vi "get_control_data.vi"(1 "DS Occurrence":refnum<k4>) -> ()   [LabVIEW 2011]
uses:
  <vilib>/Rock Robotics/WPI/Joystick/WPI_JoystickButtonState.ctl
  robot_control.ctl
  match_data.ctl
  <vilib>/Rock Robotics/WPI/DriverStation/WPI_DriverStationMatch Info.ctl
  <vilib>/Rock Robotics/WPI/DriverStation/WPI_DriverStationDerivedRobotMode.ctl
  <vilib>/Rock Robotics/WPI/DriverStation/WPI_DriverStationRobotMode.ctl
  Robot Global Data.vi
panel:
  in  "reinitialize":bool
  out "i per ms":dbl
  out "iterations":i32
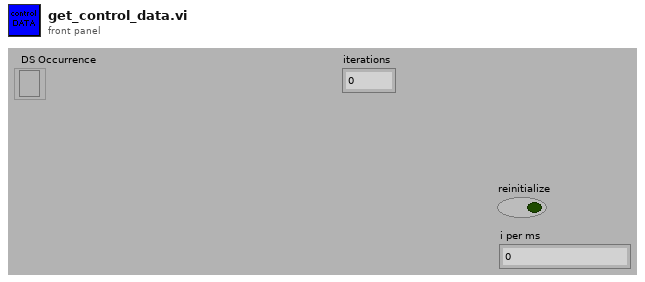
[diagram p1: front panel]
types:
  T1 = cluster{"Driver Station Digital Input (1-8)[0]":bool, "Driver Station Digital Input (1-8)[1]":bool, "Driver Station Digital Input (1-8)[2]":bool, "Driver Station Digital Input (1-8)[3]":bool, "Driver Station Digital Input (1-8)[4]":bool, "Driver Station Digital Input (1-8)[5]":bool, "Driver Station Digital Input (1-8)[6]":bool, "Driver Station Digital Input (1-8)[7]":bool, "Driver Station Digital Input (1-8)[8]":bool}
  T2 = typedef "match_data.ctl" = cluster{"Match Info":T3, "Derived Robot State":T4, "RobotMode":T5}
  T3 = typedef "WPI_DriverStationMatch Info.ctl" = cluster{"Autonomous Elapsed Seconds":dbl, "TeleOp Elapsed Seconds":dbl, "Disabled Elapsed Seconds":dbl, "Visited Autonomous":bool, "Visited TeleOp":bool, "Visited Disabled":bool, "Autonomous Settings":cluster{"Autonomous Style":enum16{"Iterative", "Independent"}, "VI Refnum":refnum<vi>}}
  T4 = typedef "WPI_DriverStationDerivedRobotMode.ctl" = enum16{"Init", "Execute", "Stop"}
  T5 = typedef "WPI_DriverStationRobotMode.ctl" = enum16{"Autonomous Disabled", "Autonomous Enabled", "Teleop Disabled", "Teleop Enabled", "Timeout", "Finish"}
  T6 = typedef "robot_control.ctl" = cluster{"Joystick1":cluster{"Buttons":T7, "Axes":cluster{"axis 1 (x)":dbl, "axis 2 (y)":dbl, "axis 3 (throttle)":dbl}}, "Joystick2":cluster{"Buttons":T7, "Axes":cluster{"axis 1 (x)":dbl, "axis 2 (y)":dbl, "axis 3 (throttle)":dbl}}, "Joystick3":cluster{"Buttons":T7, "Axes":cluster{"axis 1 (x)":dbl, "axis 2 (y)":dbl, "axis 3 (throttle)":dbl}}, "switchbox":cluster{"Driver Station Digital Input (1-8)[0]":bool, "Driver Station Digital Input (1-8)[1]":bool, "Driver Station Digital Input (1-8)[2]":bool, "Driver Station Digital Input (1-8)[3]":bool, "Driver Station Digital Input (1-8)[4]":bool, "Driver Station Digital Input (1-8)[5]":bool, "Driver Station Digital Input (1-8)[6]":bool, "Driver Station Digital Input (1-8)[7]":bool, "Driver Station Digital Input (1-8)[8]":bool}}
  T7 = typedef "WPI_JoystickButtonState.ctl" = cluster{"Button 1":bool, "Button 2":bool, "Button 3":bool, "Button 4":bool, "Button 5":bool, "Button 6":bool, "Button 7":bool, "Button 8":bool, "Button 9":bool, "Button 10":bool, "Button 11":bool, "Button 12":bool}
  T8 = cluster{"axis 1 (x)":dbl, "axis 2 (y)":dbl, "axis 3 (throttle)":dbl}
  T9 = cluster{"Buttons":T7, "Axes":cluster{"axis 1 (x)":dbl, "axis 2 (y)":dbl, "axis 3 (throttle)":dbl}}
  T10 = typedef "WPI_JoystickDevRef.ctl" = cluster{"Device":T11}
  T11 = typedef "WPI_JoystickDeviceEnum.ctl" = enum16{"USB 1", "USB 2", "USB 3", "USB 4", "Kinect 1", "Kinect 2"}
  T12 = cluster{"axis 1 (x)":dbl, "axis 2 (y)":dbl, "axis 3 (throttle)":dbl, "axis 4":dbl, "axis 5":dbl, "axis 6":dbl}
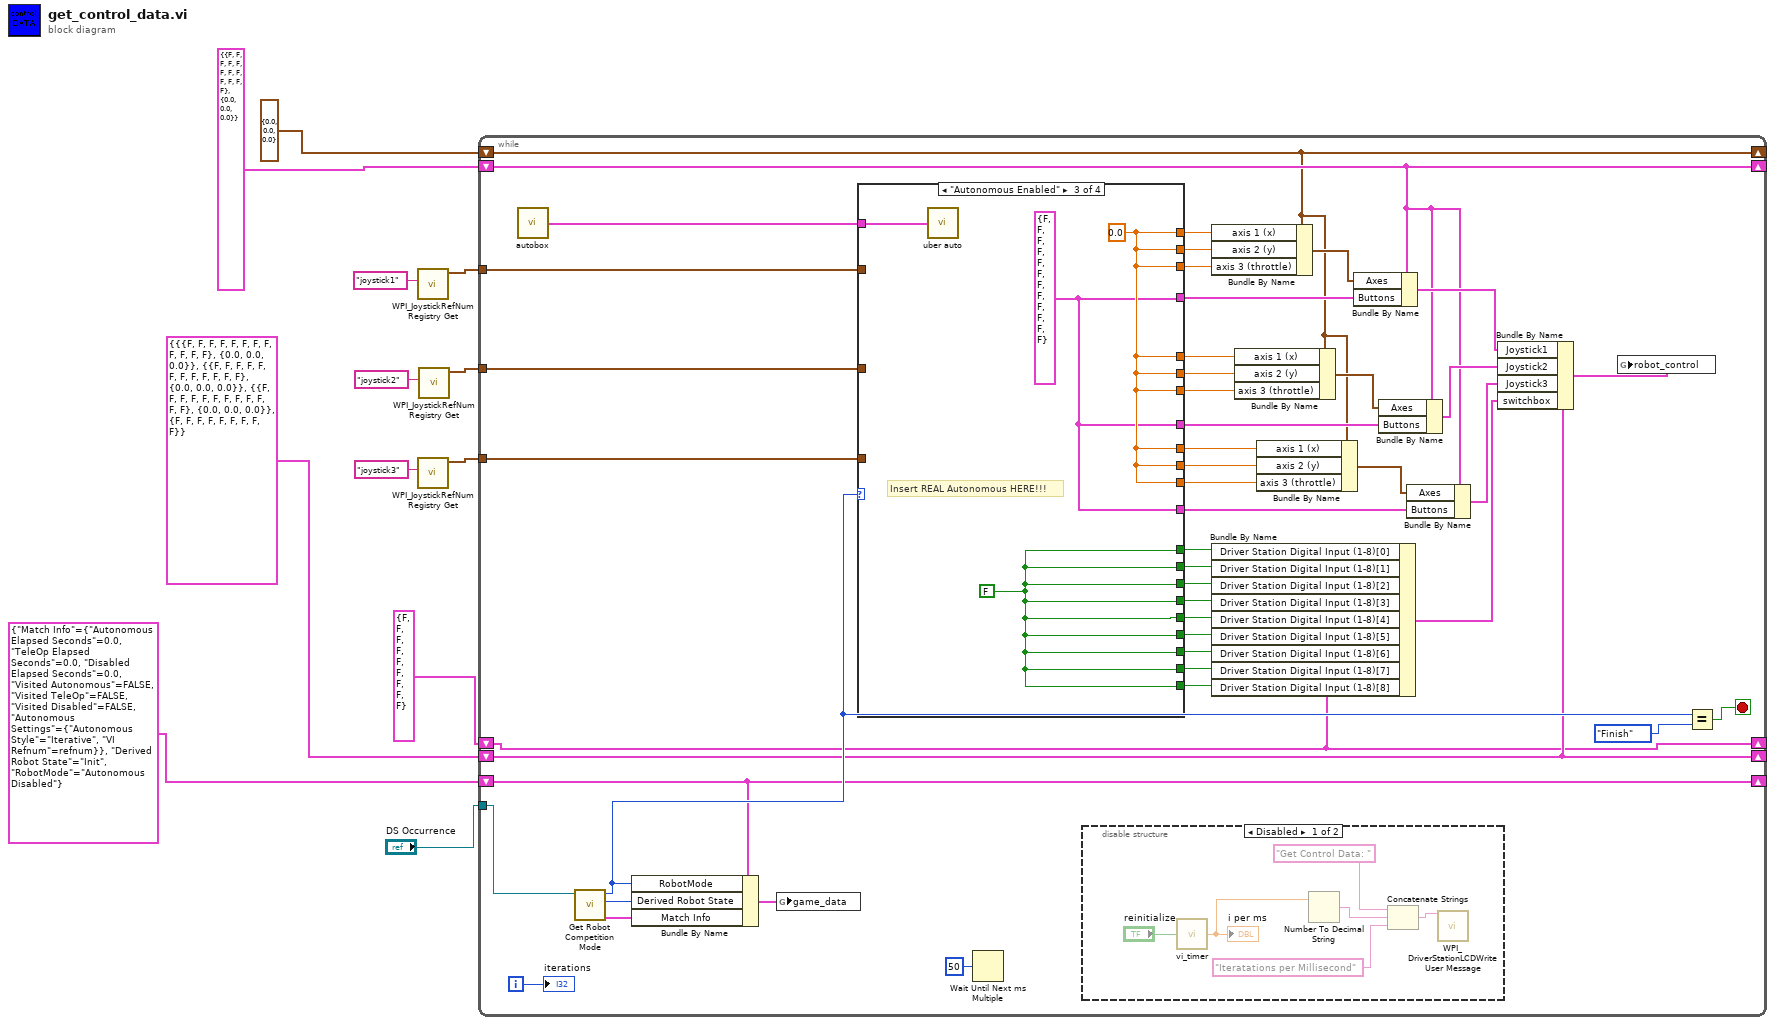
[diagram p0: block diagram]
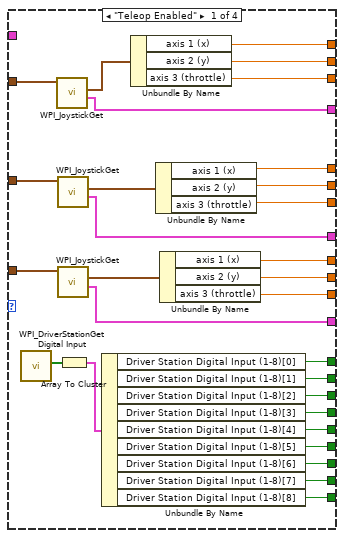
[diagram p3: hidden frame]
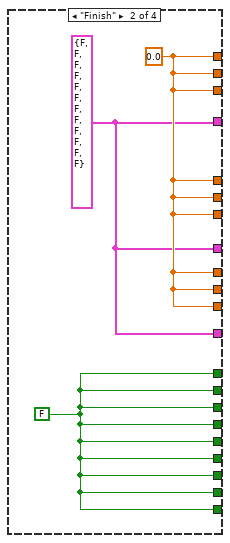
[diagram p4: hidden frame]
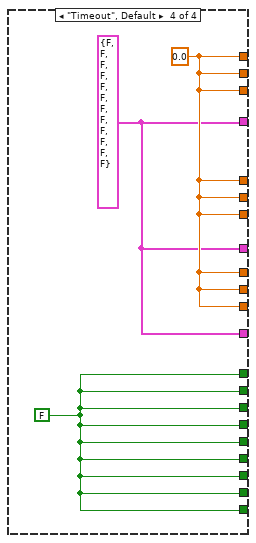
[diagram p5: hidden frame]
diagram:
  n1 = call <vilib>:"WPI_JoystickRefNum Registry Get.vi"("refnum name"="joystick1") -> ("JoystickDevRef"=w9:T10)  [unwired: 1 in, 9 out]
  n2 = call <vilib>:"WPI_JoystickRefNum Registry Get.vi"("refnum name"="joystick3") -> ("JoystickDevRef"=w11:T10)  [unwired: 1 in, 9 out]
  n3 = call <vilib>:"WPI_JoystickRefNum Registry Get.vi"("refnum name"="joystick2") -> ("JoystickDevRef"=w10:T10)  [unwired: 1 in, 9 out]
  n4 = while {
    tunnel: w11 -> [w53]
    tunnel: w10 -> [w52]
    tunnel: w9 -> [w51]
    shift-right: [w28] -> _
    shift-left: T2 {"Match Info"={"Autonomous Elapsed Seconds"=0.0, "TeleOp Elapsed Seconds"=0.0, "Disabled Elapsed Seconds"=0.0, "Visited Autonomous"=FALSE, "Visited TeleOp"=FALSE, "Visited Disabled"=FALSE, "Autonomous Settings"={"Autonomous Style"=enum."Iterative", "VI Refnum"=refnum}}, "Derived Robot State"=enum."Init", "RobotMode"=enum."Autonomous Disabled"} ("game_data") -> [w28]
    shift-right: [w29] -> _
    shift-left: T6 {"Joystick1"={"Buttons"={"Button 1"=FALSE, "Button 2"=FALSE, "Button 3"=FALSE, "Button 4"=FALSE, "Button 5"=FALSE, "Button 6"=FALSE, "Button 7"=FALSE, "Button 8"=FALSE, "Button 9"=FALSE, "Button 10"=FALSE, "Button 11"=FALSE, "Button 12"=FALSE}, "Axes"={"axis 1 (x)"=0.0, "axis 2 (y)"=0.0, "axis 3 (throttle)"=0.0}}, "Joystick2"={"Buttons"={"Button 1"=FALSE, "Button 2"=FALSE, "Button 3"=FALSE, "Button 4"=FALSE, "Button 5"=FALSE, "Button 6"=FALSE, "Button 7"=FALSE, "Button 8"=FALSE, "Button 9"=FALSE, "Button 10"=FALSE, "Button 11"=FALSE, "Button 12"=FALSE}, "Axes"={"axis 1 (x)"=0.0, "axis 2 (y)"=0.0, "axis 3 (throttle)"=0.0}}, "Joystick3"={"Buttons"={"Button 1"=FALSE, "Button 2"=FALSE, "Button 3"=FALSE, "Button 4"=FALSE, "Button 5"=FALSE, "Button 6"=FALSE, "Button 7"=FALSE, "Button 8"=FALSE, "Button 9"=FALSE, "Button 10"=FALSE, "Button 11"=FALSE, "Button 12"=FALSE}, "Axes"={"axis 1 (x)"=0.0, "axis 2 (y)"=0.0, "axis 3 (throttle)"=0.0}}, "switchbox"={"Driver Station Digital Input (1-8)[0]"=FALSE, "Driver Station Digital Input (1-8)[1]"=FALSE, "Driver Station Digital Input (1-8)[2]"=FALSE, "Driver Station Digital Input (1-8)[3]"=FALSE, "Driver Station Digital Input (1-8)[4]"=FALSE, "Driver Station Digital Input (1-8)[5]"=FALSE, "Driver Station Digital Input (1-8)[6]"=FALSE, "Driver Station Digital Input (1-8)[7]"=FALSE, "Driver Station Digital Input (1-8)[8]"=FALSE}} ("robot_control") -> [w29]
    shift-right: [w54] -> _
    shift-left: T9 {"Buttons"={"Button 1"=FALSE, "Button 2"=FALSE, "Button 3"=FALSE, "Button 4"=FALSE, "Button 5"=FALSE, "Button 6"=FALSE, "Button 7"=FALSE, "Button 8"=FALSE, "Button 9"=FALSE, "Button 10"=FALSE, "Button 11"=FALSE, "Button 12"=FALSE}, "Axes"={"axis 1 (x)"=0.0, "axis 2 (y)"=0.0, "axis 3 (throttle)"=0.0}} ("Joystick2") -> [w54]
    shift-right: [w30] -> _
    shift-left: T8 {"axis 1 (x)"=0.0, "axis 2 (y)"=0.0, "axis 3 (throttle)"=0.0} ("Axes") -> [w30]
    tunnel: "DS Occurrence" -> [w31]
    shift-right: [w24] -> _
    shift-left: T1 {"Driver Station Digital Input (1-8)[0]"=FALSE, "Driver Station Digital Input (1-8)[1]"=FALSE, "Driver Station Digital Input (1-8)[2]"=FALSE, "Driver Station Digital Input (1-8)[3]"=FALSE, "Driver Station Digital Input (1-8)[4]"=FALSE, "Driver Station Digital Input (1-8)[5]"=FALSE, "Driver Station Digital Input (1-8)[6]"=FALSE, "Driver Station Digital Input (1-8)[7]"=FALSE, "Driver Station Digital Input (1-8)[8]"=FALSE} ("switchbox") -> [w24]
    i -> [w35]
    stop <- w58 stop-if-true
    n5 = call "autobox.vi"() -> ("autobox switches"=w13:cluster{bool, bool, bool})  [unwired: 1 out]
    n6 = call "Get Robot Competition Mode.vi"("DS Occurrence"=w31) -> ("Match Info out"=w34:T3, "Call Context"=w33:T4, "Robot Mode"=w32:T5)  [unwired: 1 in, 7 out]
    n7 = Bundle By Name(cluster=w28, "RobotMode"=w32, "Derived Robot State"=w33, "Match Info"=w34) -> (w27:T2)
    n8 = global write "Robot Global Data.vi" "game_data"(w27) -> ()
    n9 = case shown="\"Autonomous Enabled\"" w32 {
      tunnel: w53 -> [w91 _ _ _]
      tunnel: w52 -> [w90 _ _ _]
      tunnel: w51 -> [w89 _ _ _]
      tunnel: [w88 w96 w100 w103] -> w50
      tunnel: [w87 w96 w100 w103] -> w49
      tunnel: [w86 w96 w100 w103] -> w48
      tunnel: [w85 w97 w101 w104] -> w47
      tunnel: [w84 w97 w101 w104] -> w46
      tunnel: [w83 w97 w101 w104] -> w45
      tunnel: [w82 w97 w101 w104] -> w44
      tunnel: [w81 w97 w101 w104] -> w43
      tunnel: [w80 w97 w101 w104] -> w42
      tunnel: [w79 w97 w101 w104] -> w41
      tunnel: [w78 w97 w101 w104] -> w40
      tunnel: [w77 w97 w101 w104] -> w39
      tunnel: [w74 w95 w99 w102] -> w23
      tunnel: [w73 w95 w99 w102] -> w22
      tunnel: [w72 w95 w99 w102] -> w21
      tunnel: [w71 w95 w99 w102] -> w20
      tunnel: [w70 w95 w99 w102] -> w19
      tunnel: [w69 w95 w99 w102] -> w18
      tunnel: [w68 w95 w99 w102] -> w17
      tunnel: [w67 w95 w99 w102] -> w16
      tunnel: [w66 w95 w99 w102] -> w15
      tunnel: w13 -> [_ _ w98 _]
      frame "Teleop Enabled" {
        n10 = call <vilib>:"WPI_DriverStationGet Digital Input.vi"() -> ("Driver Station Digital Input (1-8)"=w76:bool[])  [unwired: 11 out]
        n11 = call <vilib>:"WPI_JoystickGet.vi"("JoystickDevRef"=w89) -> ("Buttons"=w86:T7, "Axes"=w92:T12)  [unwired: 1 in, 4 out]
        n12 = call <vilib>:"WPI_JoystickGet.vi"("JoystickDevRef"=w90) -> ("Buttons"=w87:T7, "Axes"=w93:T12)  [unwired: 1 in, 4 out]
        n13 = call <vilib>:"WPI_JoystickGet.vi"("JoystickDevRef"=w91) -> ("Buttons"=w88:T7, "Axes"=w94:T12)  [unwired: 1 in, 4 out]
        n14 = Array To Cluster(array=w76) -> (cluster=w75:T1)
        n15 = Unbundle By Name(w75) -> ("Driver Station Digital Input (1-8)[0]"=w74:bool, "Driver Station Digital Input (1-8)[1]"=w73:bool, "Driver Station Digital Input (1-8)[2]"=w72:bool, "Driver Station Digital Input (1-8)[3]"=w71:bool, "Driver Station Digital Input (1-8)[4]"=w70:bool, "Driver Station Digital Input (1-8)[5]"=w69:bool, "Driver Station Digital Input (1-8)[6]"=w68:bool, "Driver Station Digital Input (1-8)[7]"=w67:bool, "Driver Station Digital Input (1-8)[8]"=w66:bool)
        n16 = Unbundle By Name(w92) -> ("axis 1 (x)"=w85:dbl, "axis 2 (y)"=w84:dbl, "axis 3 (throttle)"=w83:dbl)
        n17 = Unbundle By Name(w93) -> ("axis 1 (x)"=w82:dbl, "axis 2 (y)"=w81:dbl, "axis 3 (throttle)"=w80:dbl)
        n18 = Unbundle By Name(w94) -> ("axis 1 (x)"=w79:dbl, "axis 2 (y)"=w78:dbl, "axis 3 (throttle)"=w77:dbl)
      }
      frame "Finish" {
        w96 = T7 {"Button 1"=FALSE, "Button 2"=FALSE, "Button 3"=FALSE, "Button 4"=FALSE, "Button 5"=FALSE, "Button 6"=FALSE, "Button 7"=FALSE, "Button 8"=FALSE, "Button 9"=FALSE, "Button 10"=FALSE, "Button 11"=FALSE, "Button 12"=FALSE} ("Buttons")
        w95 = FALSE
        w97 = 0.0 ("axis 1 (x)")
      }
      frame "Autonomous Enabled" {
        w100 = T7 {"Button 1"=FALSE, "Button 2"=FALSE, "Button 3"=FALSE, "Button 4"=FALSE, "Button 5"=FALSE, "Button 6"=FALSE, "Button 7"=FALSE, "Button 8"=FALSE, "Button 9"=FALSE, "Button 10"=FALSE, "Button 11"=FALSE, "Button 12"=FALSE} ("Buttons")
        w99 = FALSE
        w101 = 0.0 ("axis 1 (x)")
        # "Insert REAL Autonomous HERE!!!"
        n19 = call "uber auto.vi"("autobox switches"=w98) -> ()  [unwired: 1 out]
      }
      frame "Timeout", Default {
        w103 = T7 {"Button 1"=FALSE, "Button 2"=FALSE, "Button 3"=FALSE, "Button 4"=FALSE, "Button 5"=FALSE, "Button 6"=FALSE, "Button 7"=FALSE, "Button 8"=FALSE, "Button 9"=FALSE, "Button 10"=FALSE, "Button 11"=FALSE, "Button 12"=FALSE} ("Buttons")
        w102 = FALSE
        w104 = 0.0 ("axis 1 (x)")
      }
    }
    n20 = Wait Until Next ms Multiple(millisecond multiple=u32 50) -> ()  [unwired: 1 out]
    n21 = disable-structure shown="Disabled" {
      frame Disabled {
        n22 = call "vi_timer.vi"("reinitialize"="reinitialize") -> ("ms/i"=w64:dbl)
        "i per ms" <- w64
        n23 = Number To Decimal String(number=w64) -> (decimal integer string=w62:string)  [unwired: 1 out]
        n24 = Concatenate Strings("Get Control Data: " ("string"), w62, "Iteratations per Millisecond" ("string")) -> (w63:string)
        n25 = call <vilib>:"WPI_DriverStationLCDWrite User Message.vi"("line text"=w63) -> ()  [unwired: 4 in, 11 out]
      }
      frame Enabled {
      }
    }
    n26 = Bundle By Name(cluster=w30, "axis 1 (x)"=w47, "axis 2 (y)"=w46, "axis 3 (throttle)"=w45) -> (w36:T8)
    n27 = Bundle By Name(cluster=w24, "Driver Station Digital Input (1-8)[0]"=w23, "Driver Station Digital Input (1-8)[1]"=w22, "Driver Station Digital Input (1-8)[2]"=w21, "Driver Station Digital Input (1-8)[3]"=w20, "Driver Station Digital Input (1-8)[4]"=w19, "Driver Station Digital Input (1-8)[5]"=w18, "Driver Station Digital Input (1-8)[6]"=w17, "Driver Station Digital Input (1-8)[7]"=w16, "Driver Station Digital Input (1-8)[8]"=w15) -> (w14:T1)
    n28 = Bundle By Name(cluster=w30, "axis 1 (x)"=w44, "axis 2 (y)"=w43, "axis 3 (throttle)"=w42) -> (w37:T8)
    n29 = Bundle By Name(cluster=w30, "axis 1 (x)"=w41, "axis 2 (y)"=w40, "axis 3 (throttle)"=w39) -> (w38:T8)
    n30 = Bundle By Name(cluster=w54, "Axes"=w36, "Buttons"=w48) -> (w57:T9)
    n31 = Bundle By Name(cluster=w54, "Axes"=w37, "Buttons"=w49) -> (w55:T9)
    n32 = Bundle By Name(cluster=w54, "Axes"=w38, "Buttons"=w50) -> (w56:T9)
    n33 = Bundle By Name(cluster=w29, "Joystick1"=w57, "Joystick2"=w55, "Joystick3"=w56, "switchbox"=w14) -> (w25:T6)
    n34 = global write "Robot Global Data.vi" "robot_control"(w25) -> ()
    n35 = Equal?(x=w32, y=WPI_DriverStationRobotMode."Finish" ("RobotMode")) -> (x = y?=w58:bool)
    "iterations" <- w35
  }
